vi "Query Marker.vi"(8 "error in (no error)":errorcluster, 10 "Marker Number":u8=1, 11 "VNA-Ag87xx in":refnum<class "VNA-Ag87xx.lvclass">) -> (0 "error out":errorcluster, 1 "Data":dbl, 2 "Frequency":dbl, 3 "VNA-Ag87xx out":refnum<class "VNA-Ag87xx.lvclass">)   [LabVIEW 2020, in "VNA-Ag87xx.lvclass"]
doc: "Query the marker on the active trace"
uses:
  VNA-Ag87xx.lvclass
  Vector Network Analyzer.lvclass
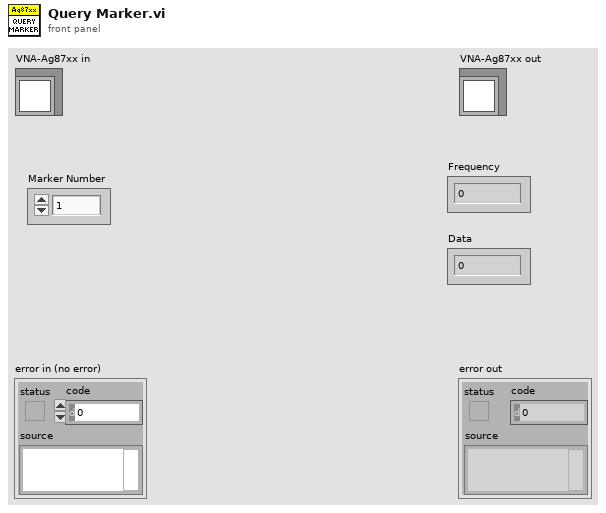
[diagram p1: front panel]
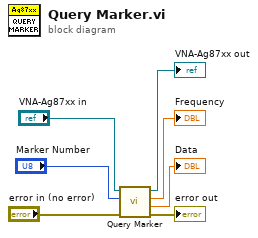
[diagram p0: block diagram]
diagram:
  n1 = call-parent "Query Marker.vi"("error in (no error)"="error in (no error)", "Marker Number"="Marker Number", "Vector Network Analyzer in"="VNA-Ag87xx in") -> ("error out"=→"error out":errorcluster, "Data"=→"Data":dbl, "Frequency"=→"Frequency":dbl, "Vector Network Analyzer out"=→"VNA-Ag87xx out":refnum<class "VNA-Ag87xx.lvclass">)  [unwired: 5 in]
